vi "Get as I64.vi"(8 "error in (no error)":errorcluster, 11 "JSON Scalar in":refnum<class "JSON Value.lvclass">) -> (0 "error out":errorcluster, 2 "Number":i64, 3 "JSON Scalar out":refnum<class "JSON Value.lvclass">)   [LabVIEW 2011, in "JSON Scalar.lvclass"]
doc: "Converts a <b>JSON Value</b> into a <b>Number</b>.\n\nCopyright 2012 James David Powell, Shaun Rumbell and Ton Plomp\nMore information on http://lavag.org/topic/16217-cr-json-labview"
uses:
  JSON Scalar.lvclass
  JSON Value/JSON Value.lvclass
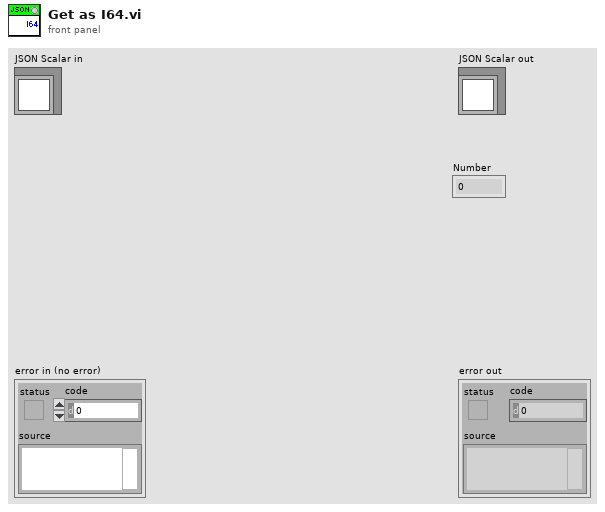
[diagram p1: front panel]
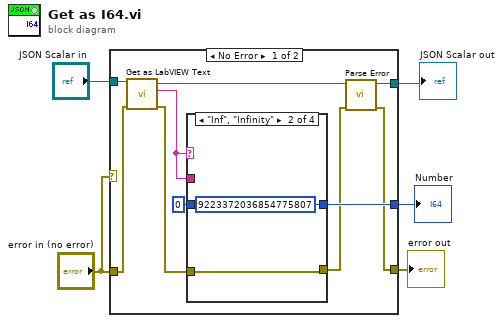
[diagram p0: block diagram]
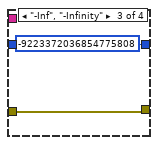
[diagram p3: hidden frame]
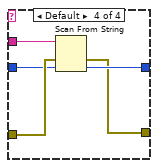
[diagram p4: hidden frame]
diagram:
  n1 = case shown="No Error" "error in (no error)" {
    tunnel: [w15 _] -> w5
    tunnel: "error in (no error)" -> [w6 w27]
    tunnel: "JSON Scalar in" -> [w13 w28]
    tunnel: [w10 w28] -> w3
    tunnel: [w8 w27] -> w2
    frame No Error {
      n2 = call-dynamic "Get as LabVIEW Text.vi"("error in (no error)"=w6, "JSON Value In"=w13) -> ("error out"=w7:errorcluster, "LabVIEW Text"=w12:string, "JSON Value Out"=w11:refnum<class "JSON Value.lvclass">)  [unwired: 7 in]
      n3 = case shown="\"Inf\", \"Infinity\"" w12 {
        tunnel: [w16 i64 9223372036854775807 ("default value 1") i64 -9223372036854775808 ("default value 1") w26] -> w15
        tunnel: w7 -> [w17 w18 w20 w25]
        tunnel: [w17 w18 w20 w24] -> w9
        tunnel: i64 0 ("default value 1") -> [w16 _ _ w23]
        tunnel: w12 -> [_ _ _ w22]
        frame "null" {
        }
        frame "Inf", "Infinity" {
        }
        frame "-Inf", "-Infinity" {
        }
        frame Default {
          n4 = Scan From String(input string=w22, error in=w25, default 1=w23) -> (error out=w24:errorcluster, output 1=w26:i64)  [unwired: 2 in, 2 out]
        }
      }
      n5 = call-dynamic "Parse Error.vi"("error in (no error)"=w9, "JSON Value in"=w11) -> ("error out"=w8:errorcluster, "JSON Value out"=w10:refnum<class "JSON Value.lvclass">)  [unwired: 8 in]
    }
    frame Error {
    }
  }
  "error out" <- w2
  "JSON Scalar out" <- w3
  "Number" <- w5
